vi "Stereo - Overlay Selected Point.vi"(7 "Group":string, 8 "error in (no error)":errorcluster, 9 "Point Coordinates":i32[](array[numeric]), 10 "Points":cluster{"X":dbl, "Y":dbl}[](array[cluster]), 11 "Image in":T1) -> (0 "error out":errorcluster, 2 "Point out":cluster{"X":dbl, "Y":dbl}, 3 "Image out":T1)   [LabVIEW 2019]
doc: "This VI locates the point closest to the Point Coordinates in the array of Points and overlays it on the image. It returns the closest point found."
uses:
  <vilib>/vision/Image Controls.llb/IMAQ Image.ctl
  <vilib>/vision/NI_Vision_Development_Module.lvlib
panel:
  # "Overview: Locates the points closest to the Point Coordinates in the array  of Points and overlays it on the image.\nThe VI also returns the closest point found."
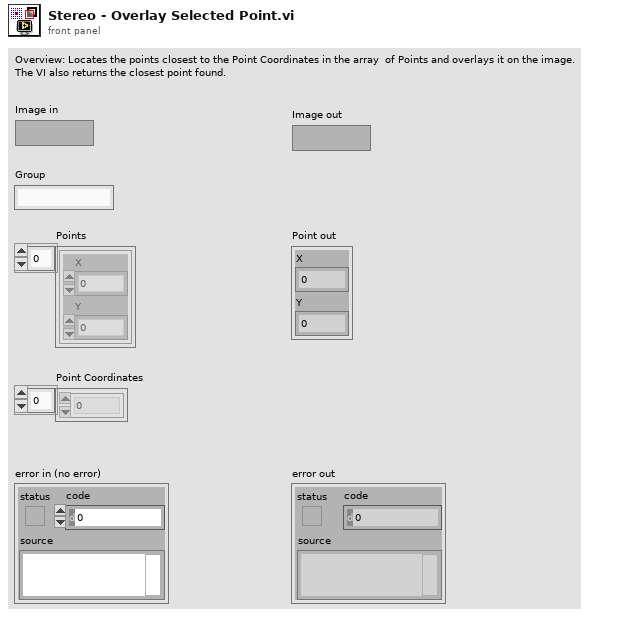
[diagram p1: front panel]
types:
  T1 = typedef "IMAQ Image.ctl" = refnum<image>
  T2 = cluster{"Point Coordinates[0]":i32, "Point Coordinates[1]":i32}
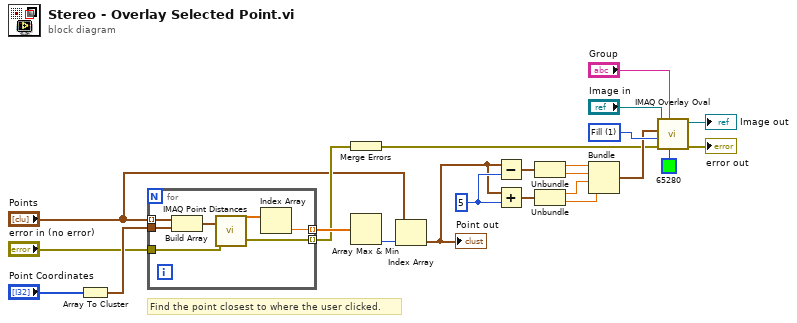
[diagram p0: block diagram]
diagram:
  w23 = 5 ("X")
  w21 = u32 1 items=["Frame", "Fill"] ("Drawing Mode (Frame)")
  # "Find the point closest to where the user clicked."
  n1 = Array To Cluster(array="Point Coordinates") -> (cluster=w13:T2)
  n2 = for {
    tunnel: "Points" -> [w30] mode=indexing
    tunnel: w13 -> [w29]
    tunnel: [w26] -> w12 mode=indexing
    tunnel: "error in (no error)" -> [w25]
    tunnel: [w24] -> w10 mode=indexing
    n3 = Build Array(w30, w29) -> (w28:cluster{"X":dbl, "Y":dbl}[])
    n4 = call "IMAQ Point Distances"("Points"=w28, "error in (no error)"=w25) -> ("Distances"=w27:sgl[], "error out"=w24:errorcluster)  [unwired: 3 out]
    n5 = Index Array(array=w27) -> (element=w26:sgl)  [unwired: 1 in]
  }
  n6 = Merge Errors(w10) -> (w9:errorcluster)
  n7 = Array Max & Min(array=w12) -> (min index (indices)=w11:i32)  [unwired: 3 out]
  n8 = Index Array(array="Points", index=w11) -> (element=w3:cluster{"X":dbl, "Y":dbl})
  "Point out" <- w3
  n9 = Subtract(x=w3, y=w23) -> (x-y=w14:cluster{"X":dbl, "Y":dbl})
  n10 = Add(x=w3, y=w23) -> (x+y=w15:cluster{"X":dbl, "Y":dbl})
  n11 = Unbundle(w14) -> ("X"=w16:dbl, "Y"=w17:dbl)
  n12 = Unbundle(w15) -> ("X"=w19:dbl, "Y"=w18:dbl)
  n13 = Bundle("X"=w16, "Y"=w17, "X"=w19, "Y"=w18) -> (w20:cluster{"X":dbl, "Y":dbl, "X":dbl, "Y":dbl})  [unwired: 1 out]
  n14 = call "IMAQ Overlay Oval"("Color"=u32 65280, "Group"="Group", "error in (no error)"=w9, "Drawing Mode (Frame)"=w21, "Bounding Rectangle"=w20, "Image"="Image in") -> ("error out"=→"error out":errorcluster, "Image Out"=→"Image out":T1)  [unwired: 4 out]
